vi "i2c_decode_status.vi"(5 "Input":T2[](array[typedef]), 7 "Relative time":bool, 9 "Initial string":string, 11 "Flag indices":i32[](array[numeric])) -> (6 "Last code string":string, 8 "Last error":bool, 10 "Result":string)   [LabVIEW 2012]
uses:
  i2c_status_cluster.ctl
  Common/i2c_status.ctl
panel:
  in  "Code":T1
  # "Visually highlight these indices"
  # "Convert from a vector of status reports to a human-readable string representation"
  # "Locals:"
  # "Just used so we can get convert from status code to string."
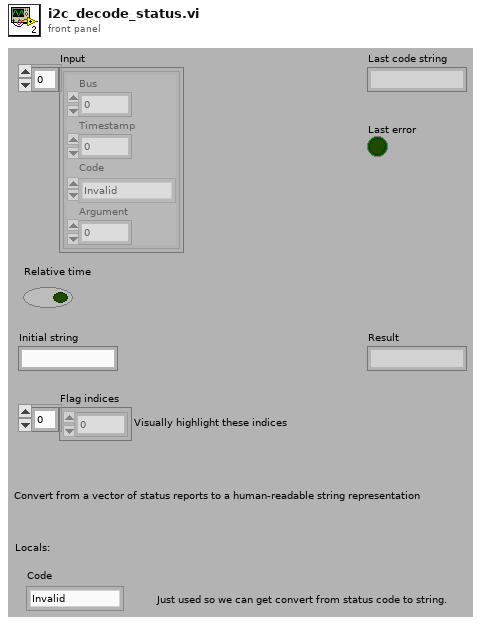
[diagram p1: front panel]
types:
  T1 = typedef "i2c_status.ctl" = enum8{"Invalid", "Command", "I2C start", "Trigger wait", "TX data wait", "Sequence", "Receive data", "I2C error", "Address NACK", "Data NACK", "SDA stuck", "SCL stuck", "Bad command"}
  T2 = typedef "i2c_status_cluster.ctl" = cluster{"Bus":u8, "Timestamp":u16, "Code":T1, "Argument":u8}
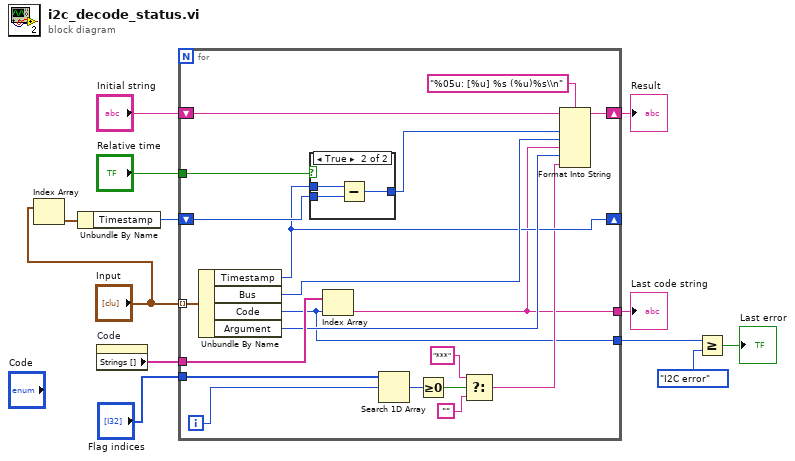
[diagram p0: block diagram]
diagram:
  n1 = Index Array(array="Input") -> (element=w9:T2)  [unwired: 1 in]
  n2 = Unbundle By Name(w9) -> ("Timestamp"=w7:u16)
  n3 = property on="Code" class="Enum (strict)"() -> ("Strings []"=w11:string[])  [unwired: 2 in, 2 out]
  n4 = for {
    tunnel: "Input" -> [w29] mode=indexing
    tunnel: w11 -> [w28]
    shift-right: [w30] -> w10
    shift-left: "Initial string" -> [w31]
    tunnel: "Relative time" -> [w25]
    shift-right: [w22] -> _
    shift-left: w7 -> [w23]
    tunnel: "Flag indices" -> [w21]
    tunnel: [w14] -> w4
    tunnel: [w13] -> w3
    i -> [w20]
    n5 = Unbundle By Name(w29) -> ("Timestamp"=w22:u16, "Bus"=w26:u8, "Code"=w13:T1, "Argument"=w27:u8)
    n6 = case shown="True" w25 {
      tunnel: w22 -> [_ w36]
      tunnel: w23 -> [w33 w35]
      tunnel: [w33 w34] -> w24
      frame False {
      }
      frame True {
        n7 = Subtract(x=w36, y=w35) -> (x-y=w34:u16)
      }
    }
    n8 = Index Array(array=w28, index=w13) -> (element=w14:string)
    n9 = Search 1D Array(1D array=w21, element=w20) -> (index of element=w19:i32)  [unwired: 1 in]
    n10 = Greater Or Equal To 0?(x=w19) -> (x >= 0?=w18:bool)
    n11 = Select(t="***", s=w18, f="") -> (s? t:f=w15:string)
    n12 = Format Into String(format string="%05u: [%u] %s (%u)%s\\n", initial string=w31, w24, w26, w14, w27, w15) -> (resulting string=w30:string)  [unwired: 1 in, 1 out]
  }
  "Result" <- w10
  "Last code string" <- w4
  n13 = Greater Or Equal?(x=w3, y=i2c_status."I2C error") -> (x >= y?=→"Last error":bool)
